vi "LCDIO Is Input On.vi"(8 "error in (no error)":errorcluster caption="Fehler (Eingang, kein Fehler)", 11 "Input Channel Handle":i64) -> (0 "error out":errorcluster caption="Fehler (Ausgang)", 3 "On":bool)   [LabVIEW 2021, in "labbCAN_DigIO_API.lvlib"]
doc: "LCDIO_Func long LCDIO_CALL LCDIO_IsInputOn(dev_hdl InChanHdl);"
uses:
  labbCAN_DigIO_API.lvlib
  labbCAN_DigIO_API.dll
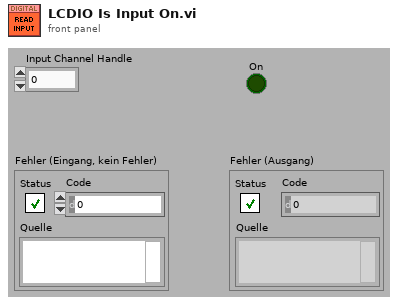
[diagram p1: front panel]
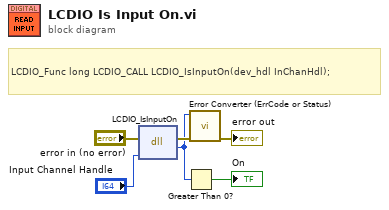
[diagram p0: block diagram]
diagram:
  # "LCDIO_Func long LCDIO_CALL LCDIO_IsInputOn(dev_hdl InChanHdl);"
  n1 = dll-call lib="C:/Users/olaja/AppData/Local/CETONI_SDK/labbCAN_DigIO_API.*" fn="LCDIO_IsInputOn"(error in="error in (no error)", "Input Channel Handle"="Input Channel Handle") -> (error out=w4:errorcluster, "Rückgabetyp"=w1:i32)  [unwired: 3 in, 1 out]
  n2 = Greater Than 0?(x=w1) -> (x > 0?=→"On":bool)
  n3 = call "Error Converter (ErrCode or Status).vi"("error in (no error)"=w4, "error code"=w1) -> ("error out"=→"error out":errorcluster)  [unwired: 9 in]
